vi "pp3_DAQ_AudioWaitStop.vi"(0 "State info":T1={"Curr  tr"=0, "Curr (ms)"=0, "Cum (ms)"=0, "Run loop diff"=0, "Tone countdown (ms)"=0, "Countdown (ms)"=0, "Curr State"=enum."15 Done", "Prev State"=enum."15 Done", "Rw"=FALSE, "Sw"=FALSE, "Tone\nGate"=FALSE, "Punish"=FALSE, "Current DAQ DO Int"=0, "Current Loaded Trial"={"Trial Type Number"=1, "Trial Type"=enum."GO", "Trial Weight"=100, "Shock (mA)"=0.3, "Duration (ms)"=0.25, "Sound Type"=enum."04 FM Sweep", "Stim P1"=4000.0, "Stim P2"=0.0, "Stim P3"=0.0, "Stim P4"=2000.0, "DAQ Amplitude (V)"=0.25}, "Next Trial (for display purposes)"={"Trial Type Number"=1, "Trial Type"=enum."GO", "Trial Weight"=100, "Shock (mA)"=0.3, "Duration (ms)"=0.25, "Sound Type"=enum."04 FM Sweep", "Stim P1"=4000.0, "Stim P2"=0.0, "Stim P3"=0.0, "Stim P4"=2000.0, "DAQ Amplitude (V)"=0.25}, "Total trials memo"=0, "State start cum memo (ms)"=0, "Last dur jump time memo (ms)"=0, "Last dur shock time memo (ms)"=0, "Tone repeat memo (ms)"=0, "Webcam on"=FALSE, "Webcam recording"=FALSE, "State update flag"=FALSE, "Last loaded shock voltage"=0.0, "Vid upd"=enum."0"} {"Current DAQ DO Int" format="%016b"; "Next Trial (for display purposes)"."DAQ Amplitude (V)" min=0.0 max=5.0 format="%_6g"; "Next Trial (for display purposes)"."Shock (mA)" min=-1.0 max=5.0; "Next Trial (for display purposes)"."Trial Weight" step=1; "Next Trial (for display purposes)"."Duration (ms)" min=0.0 max=1.0; "Next Trial (for display purposes)"."Trial Type Number" min=1 max=256 step=1; "Current Loaded Trial"."DAQ Amplitude (V)" min=0.0 max=5.0 format="%_6g"; "Current Loaded Trial"."Shock (mA)" min=-1.0 max=5.0; "Current Loaded Trial"."Trial Weight" step=1; "Current Loaded Trial"."Duration (ms)" min=0.0 max=1.0; "Current Loaded Trial"."Trial Type Number" min=1 max=256 step=1}, 5 "Daq config In":T6={"Sound AO"="Dev2/ao0", "Shock intesity AO"="Dev1/ao1", "Code_LED DO"="Dev1/port1:2", "Switch DI"="Dev1/port0/line0:1", "Webcam"="cam0", "Sound AO task"="", "Sound card task"=0, "Shock intensity AO task"="", "Code_LED DO task"="", "Switch DI task"="", "AO <=> Sound card"=FALSE, "Sound card"=0, "sample rate"=8000.0, "Variable shock"=FALSE, "Webcam on"=FALSE, "Tone gate PFI"="/Dev1/PFI1", "Waveform memo"={"t0"=timestamp(0 s since 1904-01-01), "dt"=1.0, "Y"=[]}, "First time"=FALSE} {"sample rate" min=8000.0; "Sound card task" format="%.0x"}, 11 "error in (no error)":errorcluster) -> (4 "State info out":T1={"Curr  tr"=0, "Curr (ms)"=0, "Cum (ms)"=0, "Run loop diff"=0, "Tone countdown (ms)"=0, "Countdown (ms)"=0, "Curr State"=enum."15 Done", "Prev State"=enum."15 Done", "Rw"=FALSE, "Sw"=FALSE, "Tone\nGate"=FALSE, "Punish"=FALSE, "Current DAQ DO Int"=0, "Current Loaded Trial"={"Trial Type Number"=1, "Trial Type"=enum."GO", "Trial Weight"=100, "Shock (mA)"=0.3, "Duration (ms)"=0.25, "Sound Type"=enum."04 FM Sweep", "Stim P1"=4000.0, "Stim P2"=0.0, "Stim P3"=0.0, "Stim P4"=2000.0, "DAQ Amplitude (V)"=0.25}, "Next Trial (for display purposes)"={"Trial Type Number"=1, "Trial Type"=enum."GO", "Trial Weight"=100, "Shock (mA)"=0.3, "Duration (ms)"=0.25, "Sound Type"=enum."04 FM Sweep", "Stim P1"=4000.0, "Stim P2"=0.0, "Stim P3"=0.0, "Stim P4"=2000.0, "DAQ Amplitude (V)"=0.25}, "Total trials memo"=0, "State start cum memo (ms)"=0, "Last dur jump time memo (ms)"=0, "Last dur shock time memo (ms)"=0, "Tone repeat memo (ms)"=0, "Webcam on"=FALSE, "Webcam recording"=FALSE, "State update flag"=FALSE, "Last loaded shock voltage"=0.0, "Vid upd"=enum."0"} {"Current DAQ DO Int" format="%016b"; "Next Trial (for display purposes)"."DAQ Amplitude (V)" min=0.0 max=5.0 format="%_6g"; "Next Trial (for display purposes)"."Shock (mA)" min=-1.0 max=5.0; "Next Trial (for display purposes)"."Trial Weight" step=1; "Next Trial (for display purposes)"."Duration (ms)" min=0.0 max=1.0; "Next Trial (for display purposes)"."Trial Type Number" min=1 max=256 step=1; "Current Loaded Trial"."DAQ Amplitude (V)" min=0.0 max=5.0 format="%_6g"; "Current Loaded Trial"."Shock (mA)" min=-1.0 max=5.0; "Current Loaded Trial"."Trial Weight" step=1; "Current Loaded Trial"."Duration (ms)" min=0.0 max=1.0; "Current Loaded Trial"."Trial Type Number" min=1 max=256 step=1}, 6 "Daq config Out":T6={"Sound AO"="Dev2/ao0", "Shock intesity AO"="Dev1/ao1", "Code_LED DO"="Dev1/port1:2", "Switch DI"="Dev1/port0/line0:1", "Webcam"="cam0", "Sound AO task"="", "Sound card task"=0, "Shock intensity AO task"="", "Code_LED DO task"="", "Switch DI task"="", "AO <=> Sound card"=FALSE, "Sound card"=0, "sample rate"=8000.0, "Variable shock"=FALSE, "Webcam on"=FALSE, "Tone gate PFI"="/Dev1/PFI1", "Waveform memo"={"t0"=timestamp(0 s since 1904-01-01), "dt"=1.0, "Y"=[]}, "First time"=FALSE} {"sample rate" min=8000.0; "Sound card task" format="%.0x"}, 15 "error out":errorcluster)   [LabVIEW 2013]
uses:
  pp2_CTL_DaqConfig.ctl
  <vilib>/userdefined/High Color/IMAQdx.ctl
  <vilib>/sound2/lvsound2.llb/Sound Output Task ID.ctl
  pp3_CTL_StateInfo.ctl
  pp3_CTL_State.ctl
  pp3_CTL_Trial.ctl
  pp3_CTL_TrialType.ctl
  labolabo2/waveforms/WFTypes.ctl
  <resource>/objmgr/daqmx.rc
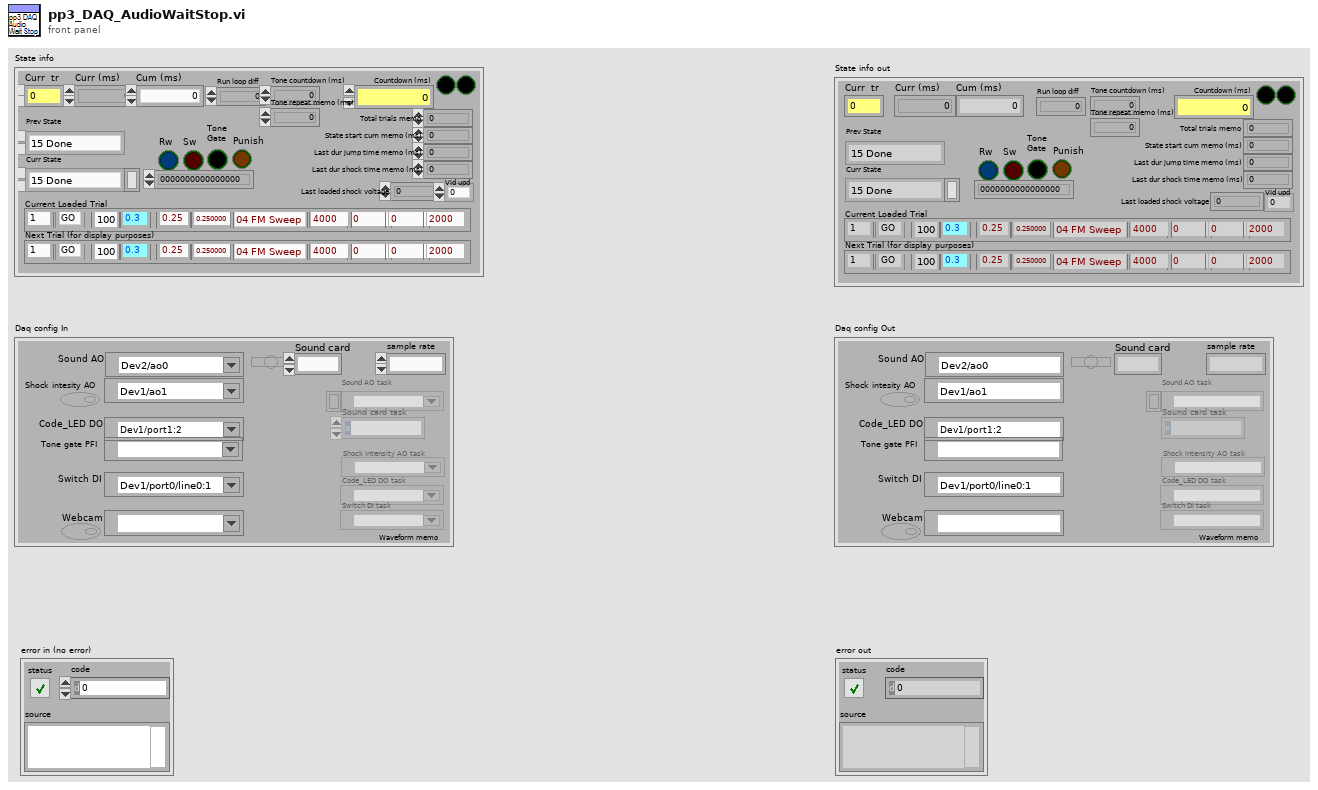
[diagram p1: front panel]
types:
  T1 = typedef "pp3_CTL_StateInfo.ctl" = cluster{"Curr  tr":u16, "Curr (ms)":u32, "Cum (ms)":i64, "Run loop diff":i64, "Tone countdown (ms)":i64, "Countdown (ms)":i64, "Curr State":T2, "Prev State":T2, "Rw":bool, "Sw":bool, "Tone\nGate":bool, "Punish":bool, "Current DAQ DO Int":u16, "Current Loaded Trial":T3, "Next Trial (for display purposes)":T3, "Total trials memo":i64, "State start cum memo (ms)":i64, "Last dur jump time memo (ms)":i64, "Last dur shock time memo (ms)":i64, "Tone repeat memo (ms)":i64, "Webcam on":bool, "Webcam recording":bool, "State update flag":bool, "Last loaded shock voltage":dbl, "Vid upd":enum16{"0", "1", "2", "3", "4", "5", "6", "7", "8", "9"}}
  T2 = typedef "pp3_CTL_State.ctl" = enum8{"0 NULL", "1 Habituation", "2 (Load Trial)", "3 Stay Period", "4 Load Audio/Click Delay", "5 GO Trial", "6 GO Jumped", "7 GO Timeout", "8 NOGO Trial", "9 NOGO Jumped", "10 NOGO Timeout", "11 TEST Trial", "12 TEST Jumped", "13 TEST Timeout", "14 Intertrial Interval", "15 Done"}
  T3 = typedef "pp3_CTL_Trial.ctl" = cluster{"Trial Type Number":i16, "Trial Type":T4, "Trial Weight":u32, "Shock (mA)":dbl, "Duration (ms)":dbl, "Sound Type":T5, "Stim P1":dbl, "Stim P2":dbl, "Stim P3":dbl, "Stim P4":dbl, "DAQ Amplitude (V)":dbl}
  T4 = typedef "pp3_CTL_TrialType.ctl" = enum16{"OFF", "GO", "NOGO", "TEST"}
  T5 = typedef "WFTypes.ctl" = enum16{"00 NULL", "01 DC", "02 Noise", "03 Pure Tone", "04 FM Sweep"}
  T6 = typedef "pp2_CTL_DaqConfig.ctl" = cluster{"Sound AO":tag, "Shock intesity AO":tag, "Code_LED DO":tag, "Switch DI":tag, "Webcam":T7, "Sound AO task":refnum<k21>, "Sound card task":T8, "Shock intensity AO task":refnum<k21>, "Code_LED DO task":refnum<k21>, "Switch DI task":refnum<k21>, "AO <=> Sound card":bool, "Sound card":u32, "sample rate":dbl, "Variable shock":bool, "Webcam on":bool, "Tone gate PFI":tag, "Waveform memo":waveform(dbl), "First time":bool}
  T7 = typedef "IMAQdx.ctl" = refnum<k21>
  T8 = typedef "Sound Output Task ID.ctl" = u32
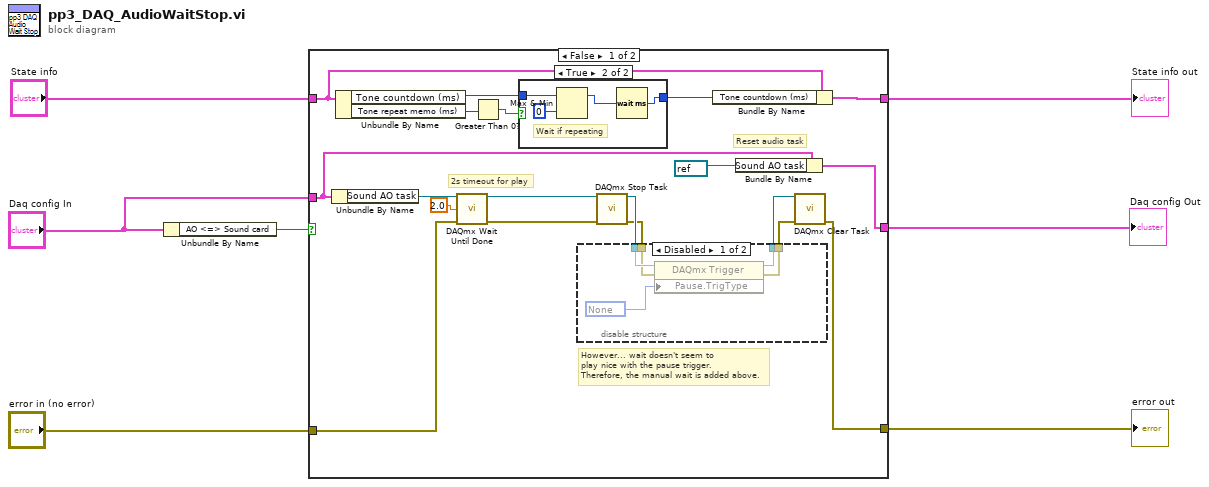
[diagram p0: block diagram]
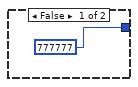
[diagram p2: hidden frame]
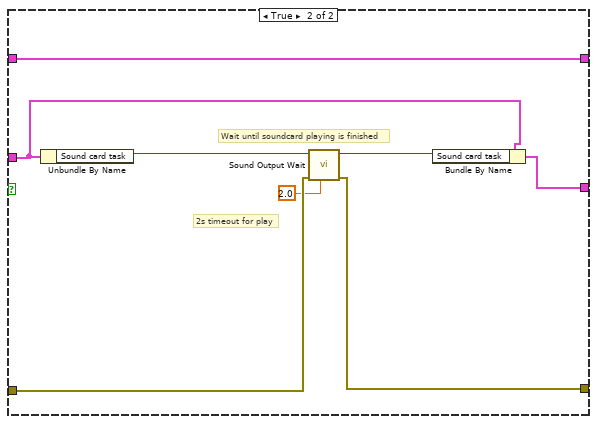
[diagram p4: hidden frame]
diagram:
  n1 = Unbundle By Name("Daq config In") -> ("AO <=> Sound card"=w5:bool)
  n2 = case shown="False" w5 {
    tunnel: "error in (no error)" -> [w26 w46]
    tunnel: [w11 w45] -> w6
    tunnel: "Daq config In" -> [w14 w40]
    tunnel: "State info" -> [w22 w44]
    tunnel: [w21 w44] -> w2
    tunnel: [w12 w41] -> w1
    frame False {
      # "Reset audio task"
      # "However... wait doesn't seem to\nplay nice with the pause trigger.\nTherefore, the manual wait is added above."
      # "2s timeout for play"
      n3 = Unbundle By Name(w14) -> ("Sound AO task"=w24:refnum<k21>)
      n4 = Unbundle By Name(w22) -> ("Tone countdown (ms)"=w23:i64, "Tone repeat memo (ms)"=w10:i64)
      n5 = call <vilib>:"DAQmx Wait Until Done.vi"("task/channels in"=w24, "timeout (sec)"=2.0 ("timeout"), "error in"=w26) -> ("task out"=w16:refnum<k21>, "error out"=w15:errorcluster)  [unwired: 11 in]
      n6 = Greater Than 0?(x=w10) -> (x > 0?=w9:bool)
      n7 = case shown="True" w9 {
        tunnel: w23 -> [_ w31]
        tunnel: [i64 777777 ("Countdown (ms)") w28] -> w8
        frame False {
        }
        frame True {
          # "Wait if repeating"
          n8 = Max & Min(x=w31, y=i64 0) -> (max(x,y)=w29:i64)  [unwired: 1 out]
          n9 = Wait (ms)(milliseconds to wait=w29) -> (millisecond timer value=w28:u32)
        }
      }
      n10 = call <vilib>:"DAQmx Stop Task.vi"("task/channels in"=w16, "error in"=w15) -> ("task out"=w20:refnum<k21>, "error out"=w19:errorcluster)  [unwired: 12 in]
      n11 = disable-structure shown="Disabled" {
        disable-tunnel: w20 -> [w36 w38]
        disable-tunnel: w19 -> [w35 w37]
        disable-tunnel: [w34 w38] -> w18
        disable-tunnel: [w33 w37] -> w17
        frame Disabled {
          w32 = 10230 items=["Analog Level"=10101, "Analog Window"=10103, "Digital Level"=10152, "Digital Pattern"=10398, "None"=10230] ("Pause.TrigType")
          n12 = property class="DAQmx Trigger"(reference=w36, error in=w35, "Pause.TrigType"=w32) -> (reference out=w34:refnum<k21>, error out=w33:errorcluster)
        }
        frame Enabled {
        }
      }
      n13 = Bundle By Name(cluster=w22, "Tone countdown (ms)"=w8) -> (w21:T1)
      n14 = Bundle By Name(cluster=w14, "Sound AO task"=refnum<k21> refnum) -> (w12:T6)
      n15 = call <vilib>:"DAQmx Clear Task.vi"("task in"=w18, "error in"=w17) -> ("error out"=w11:errorcluster)  [unwired: 13 in]
    }
    frame True {
      # "2s timeout for play"
      # "Wait until soundcard playing is finished"
      n16 = Unbundle By Name(w40) -> ("Sound card task"=w42:T8)
      n17 = call <vilib>:"Sound Output Wait.vi"("timeout (sec)"=2.0, "error in (no error)"=w46, "task ID"=w42) -> ("error out"=w45:errorcluster, "task ID out"=w43:T8)  [unwired: 7 in]
      n18 = Bundle By Name(cluster=w40, "Sound card task"=w43) -> (w41:T6)
    }
  }
  "Daq config Out" <- w1
  "error out" <- w6
  "State info out" <- w2
